vi "niFpga wdp fft apply twid factors dummy.vi"(6 "enable":bool, 8 "data index 1":fxp<+,9,9>, 9 "data index 0":fxp<+,9,9>, 10 "data in 1":T1(array[cluster])=[{"data re"=0.0, "data im"=0.0}, {"data re"=0.0, "data im"=0.0}, {"data re"=0.0, "data im"=0.0}, {"data re"=0.0, "data im"=0.0}, {"data re"=0.0, "data im"=0.0}, {"data re"=0.0, "data im"=0.0}, {"data re"=0.0, "data im"=0.0}, {"data re"=0.0, "data im"=0.0}], 11 "data in 0":T1(array[cluster])=[{"data re"=0.0, "data im"=0.0}, {"data re"=0.0, "data im"=0.0}, {"data re"=0.0, "data im"=0.0}, {"data re"=0.0, "data im"=0.0}, {"data re"=0.0, "data im"=0.0}, {"data re"=0.0, "data im"=0.0}, {"data re"=0.0, "data im"=0.0}, {"data re"=0.0, "data im"=0.0}]) -> (2 "data out 1":T1(array[cluster]), 3 "data out 0":T1(array[cluster]))   [LabVIEW 2017]
types:
  T1 = cluster{"data re":fxp<+/-,8,1>, "data im":fxp<+/-,8,1>}[]
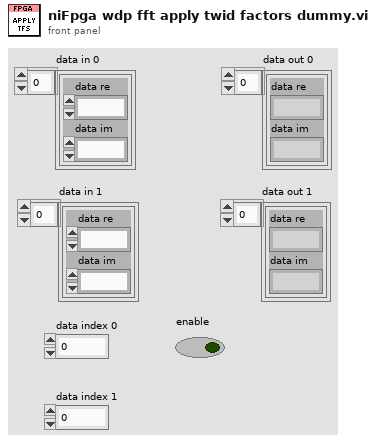
[diagram p1: front panel]
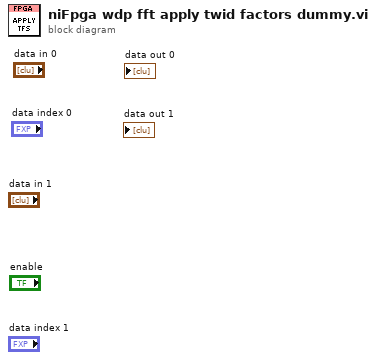
[diagram p0: block diagram]
diagram:
